vi "Main.vi"() -> ()   [LabVIEW 2024]
uses:
  <vilib>/userDefined/High Color/IMAQdx.ctl
  <vilib>/vision/Image Controls.llb/IMAQ Image.ctl
  <vilib>/vision/driver/NI_Vision_Acquisition_Software.lvlib
panel:
  in  "Exit Application":bool caption="Click to terminate the application"
  in  "Tab Control":enum32{"Page 1", "Page 2", "Page 3", "Page 4"}(tab)
  in  "OK Button":bool
  out "Image Display":T1(plugin-control)
  in  "Settings Button":bool
  in  "Add user":bool
  out "Current VI":path
  in  "Back to userpage":bool
  out "Image Display 2":T1(plugin-control)
  in  "OK Button 2":bool
  in  "String":string
  in  "String 2":string
  # "Processing..."
  # "Welcome to control panel"
  # "Now you can chose what you want to do"
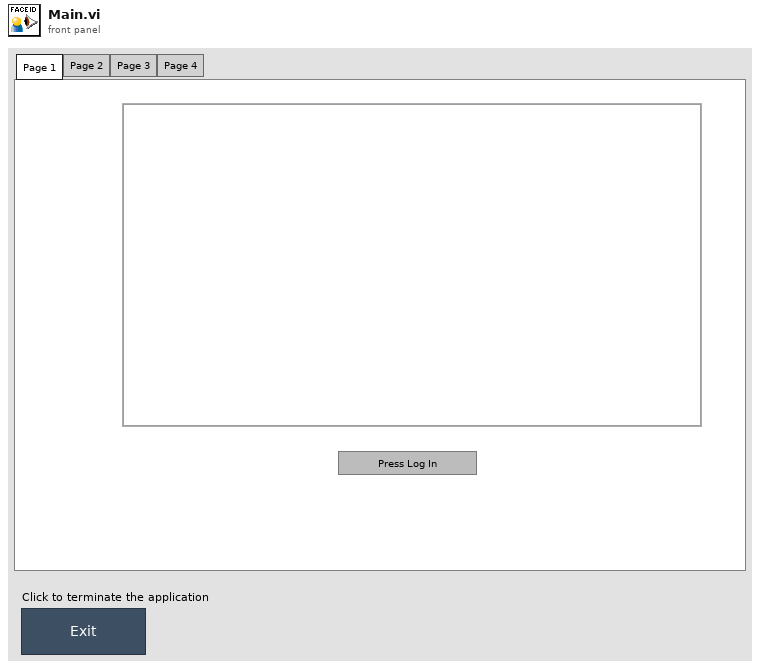
[diagram p1: front panel]
types:
  T1 = typedef "IMAQ Image.ctl" = refnum<image>
  T2 = enum32{"Invalid", "Standard", "Closed", "Hidden", "Minimized", "Maximized"}
  T3 = enum32{"invalid app kind", "Development System", "Run Time System", "Student Edition", "Embedded LabVIEW", "Evaluation", "Custom"}
  T4 = typedef "IMAQdx.ctl" = refnum<k21>
  T5 = cluster{"Core":cluster{"Current VI Reference":refnum<vi>, "Close Panel on Exit?":bool}, "New Image":T1, "IMAQdx Session":T4, "Img Path":string}
  T6 = cluster{"Current VI Reference":refnum<vi>, "Close Panel on Exit?":bool}
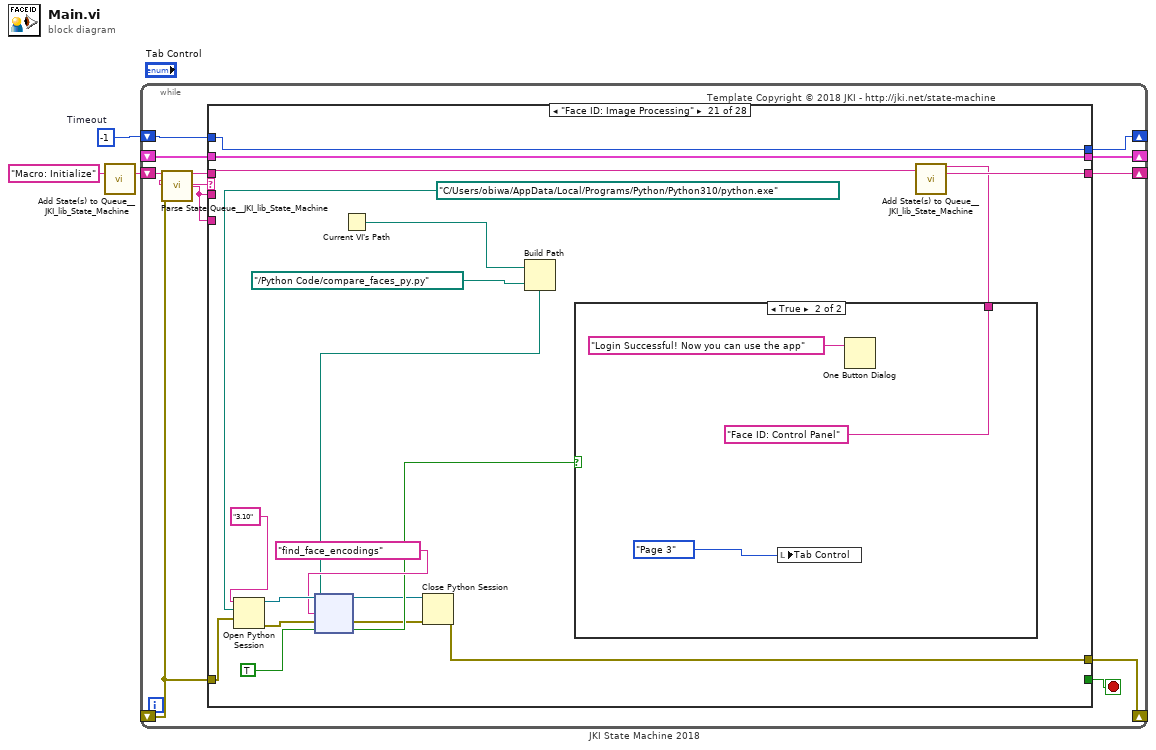
[diagram p0: block diagram]
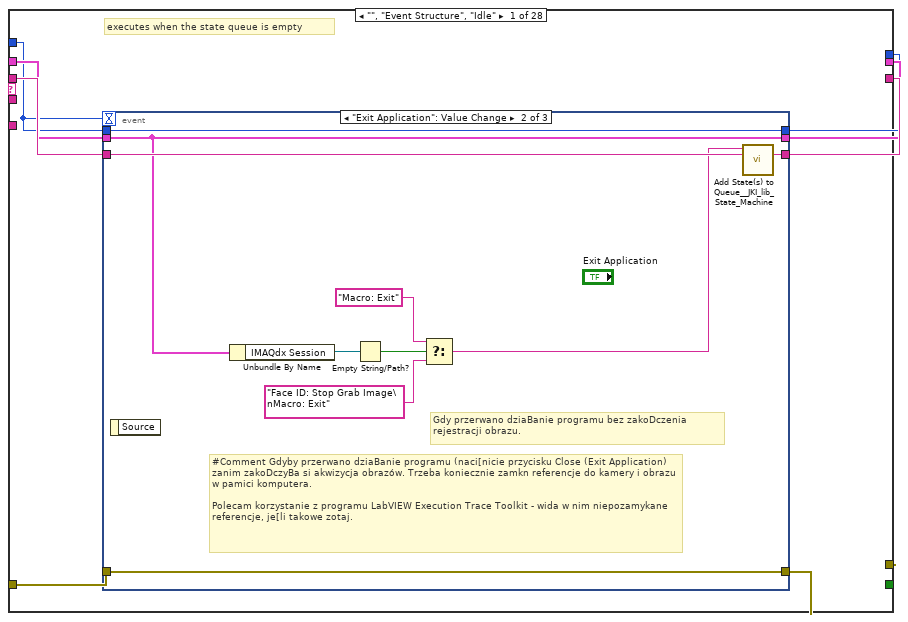
[diagram p2: hidden frame]
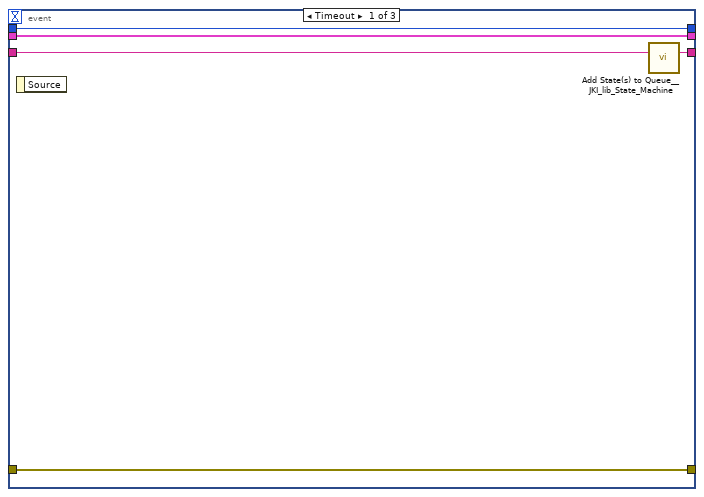
[diagram p3: hidden frame]
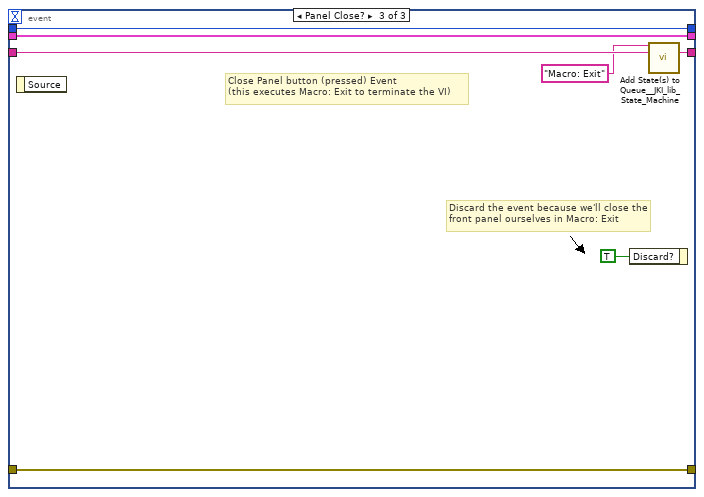
[diagram p4: hidden frame]
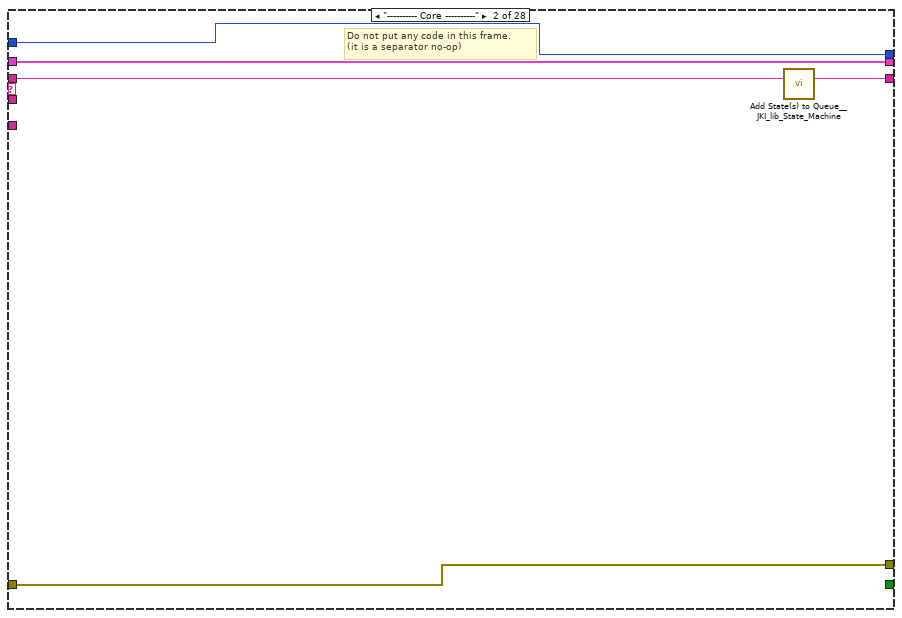
[diagram p5: hidden frame]
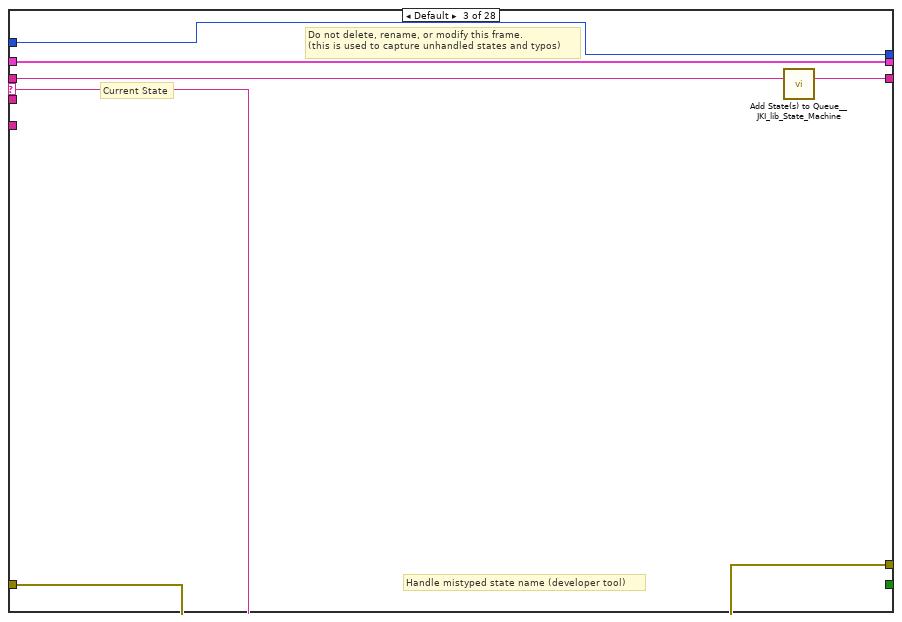
[diagram p6: hidden frame]
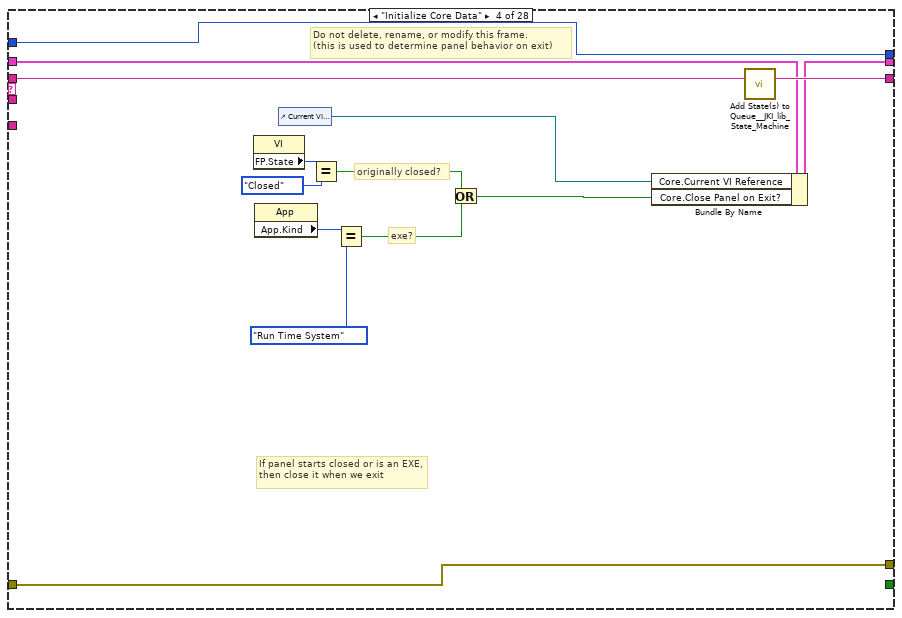
[diagram p7: hidden frame]
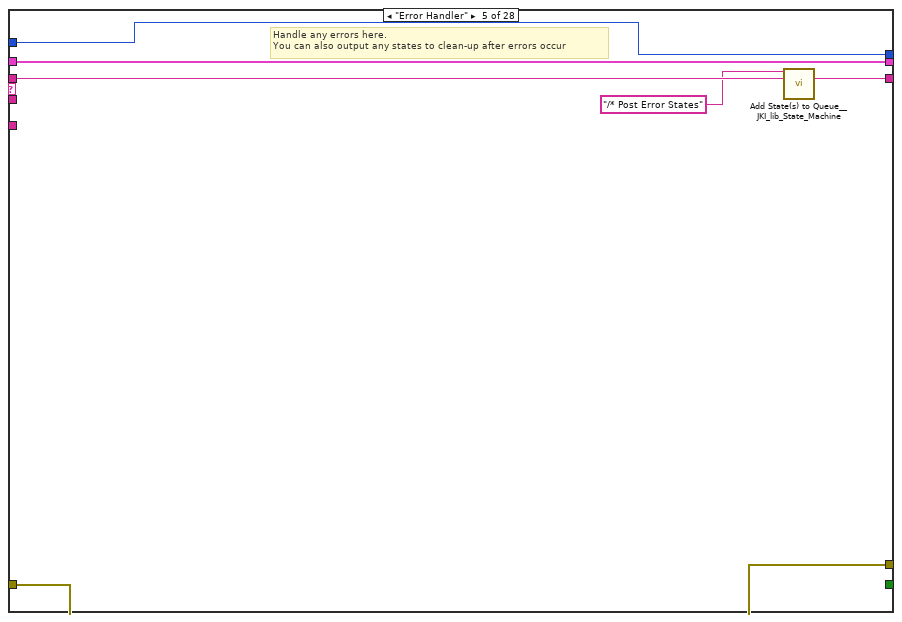
[diagram p8: hidden frame]
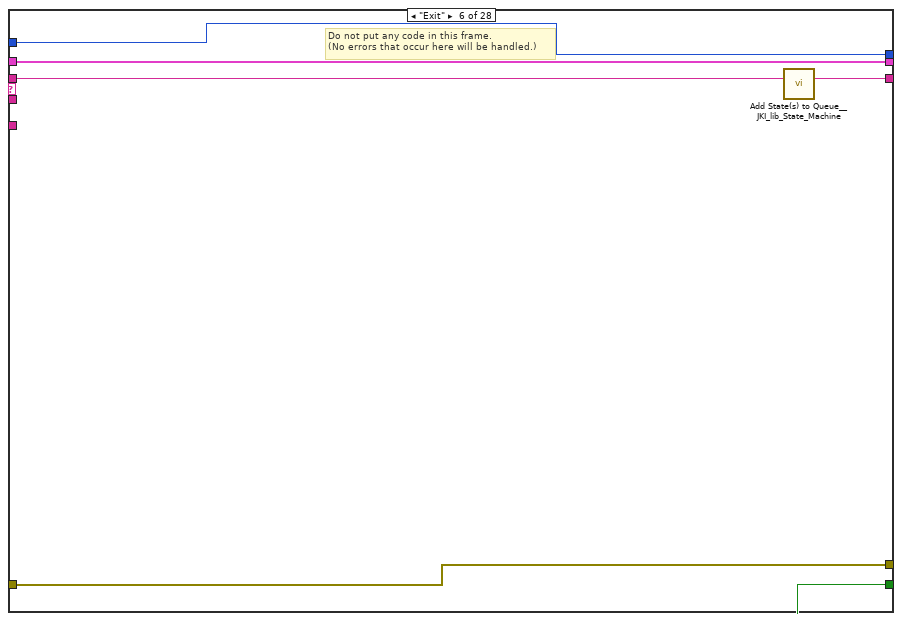
[diagram p9: hidden frame]
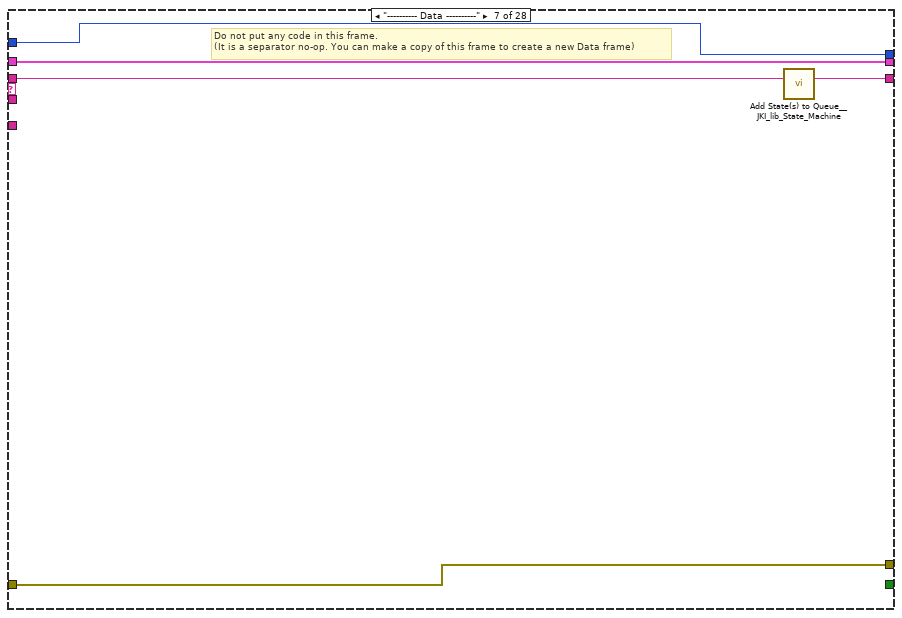
[diagram p10: hidden frame]
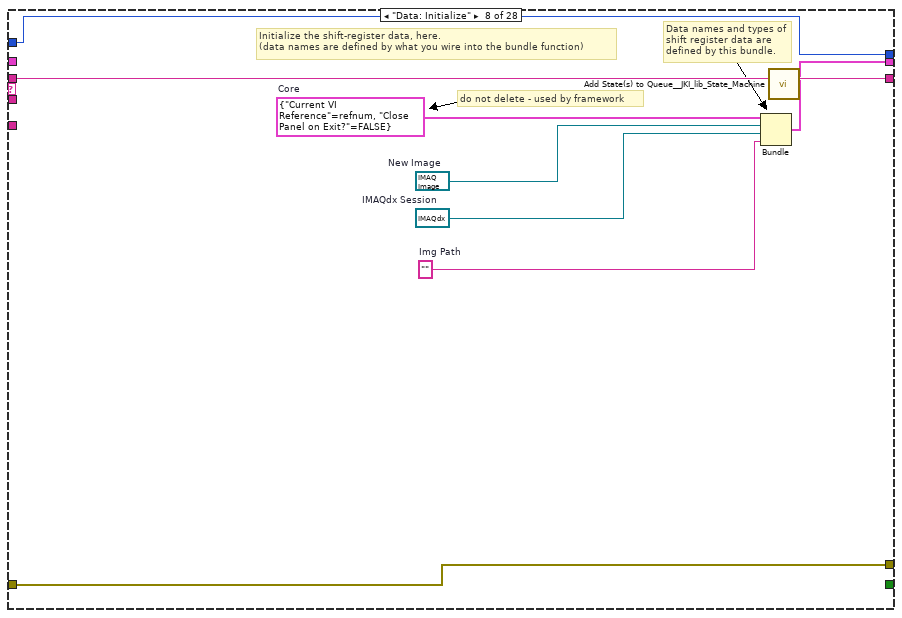
[diagram p11: hidden frame]
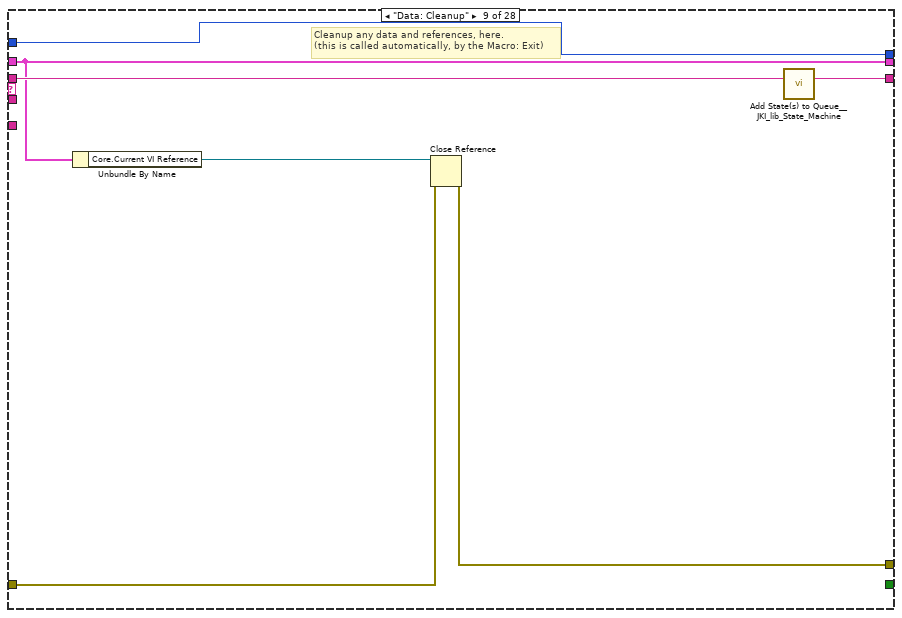
[diagram p12: hidden frame]
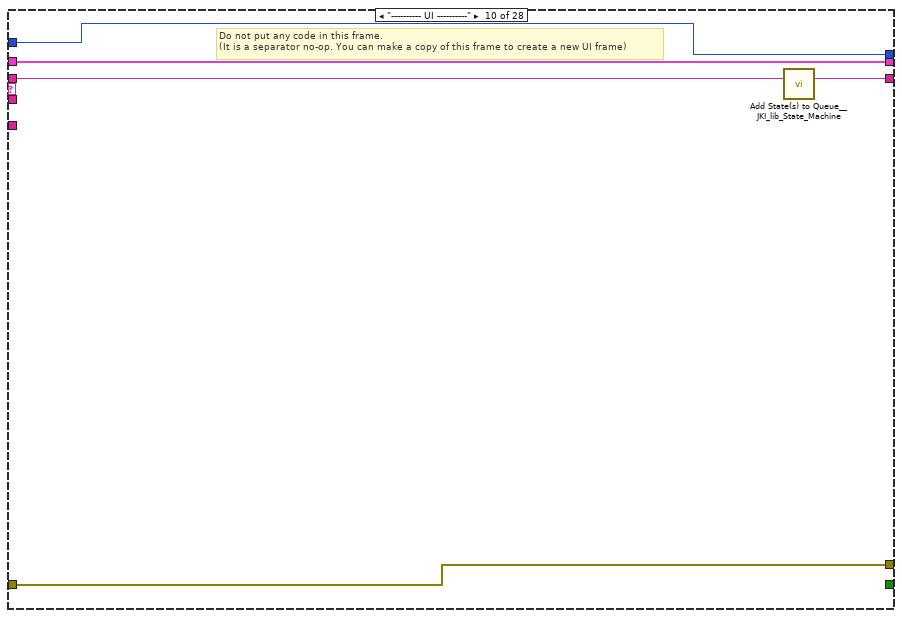
[diagram p13: hidden frame]
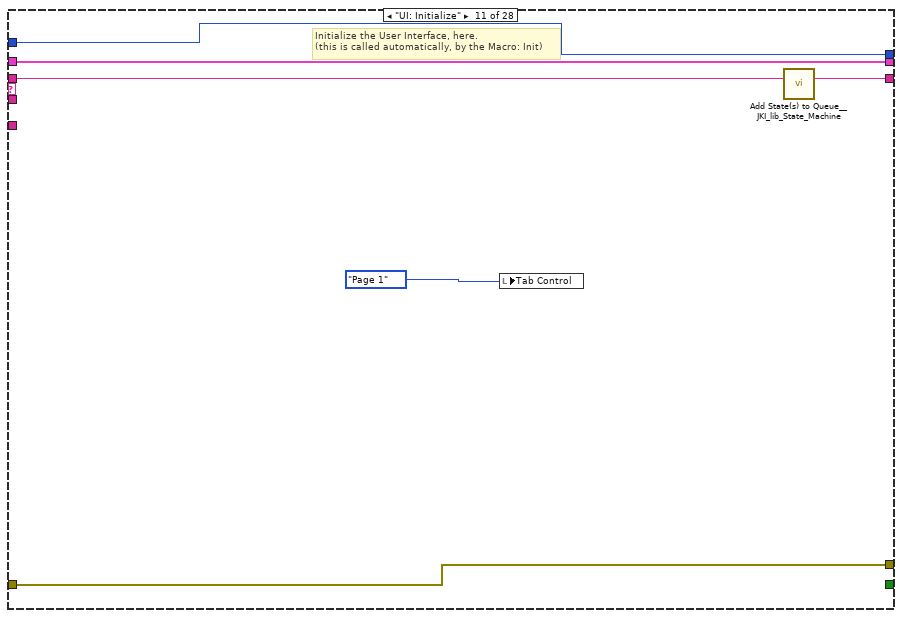
[diagram p14: hidden frame]
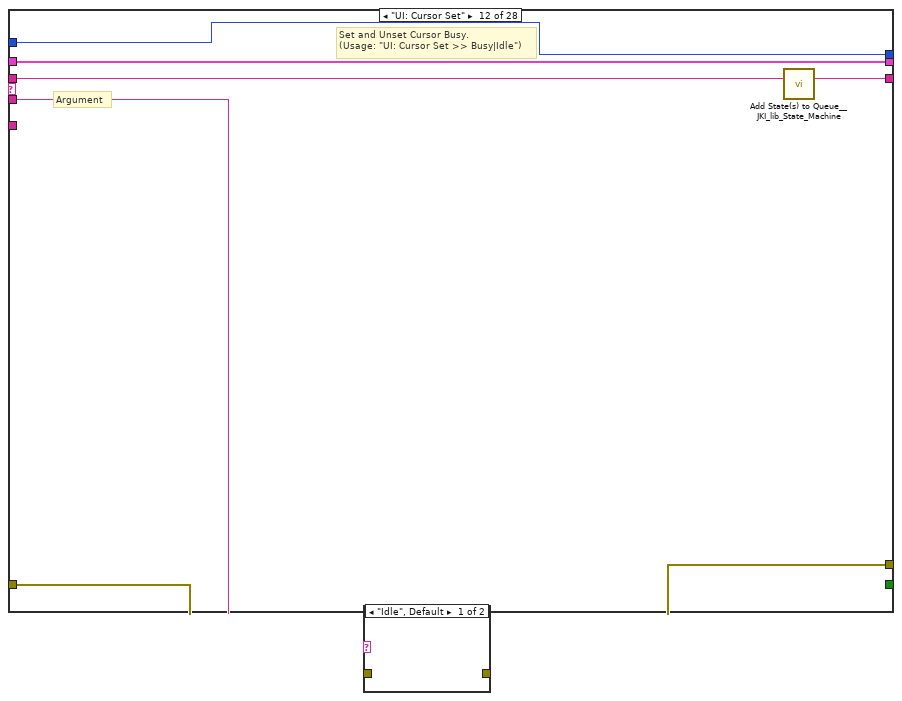
[diagram p15: hidden frame]
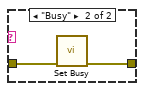
[diagram p16: hidden frame]
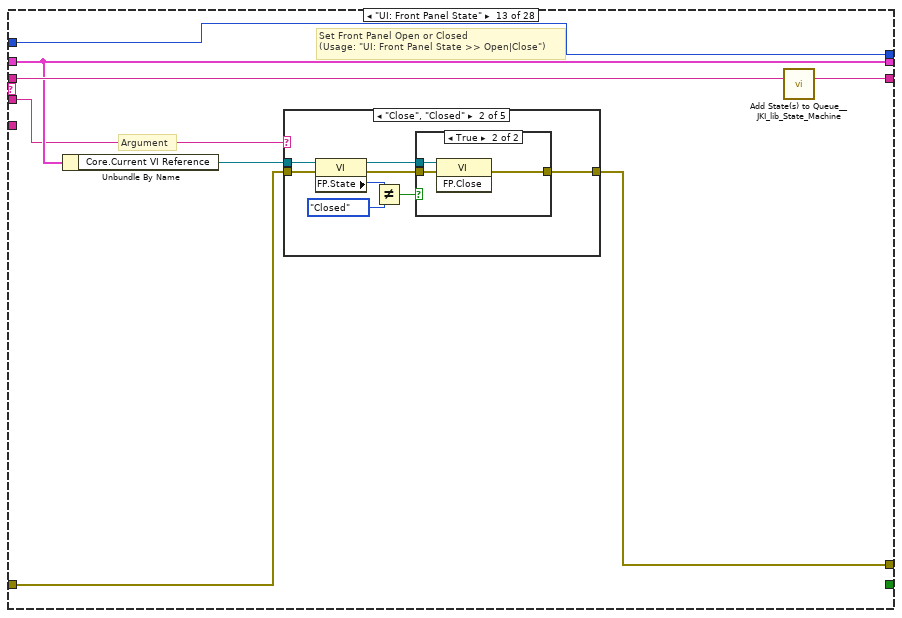
[diagram p17: hidden frame]
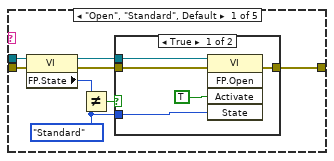
[diagram p18: hidden frame]
diagram:
  w1 = -1  # Timeout
  n1 = call <vilib>:"Add State(s) to Queue__JKI_lib_State_Machine.vi"("State(s) in (\"\")"="Macro: Initialize") -> ("States Out"=w3:string)  [unwired: 14 in]
  n2 = while "JKI State Machine 2018" {
    shift-right: [w9] -> _
    shift-left: _ -> [w8]
    shift-right: [w12] -> _
    shift-left: _ -> [w7]
    shift-right: [w11] -> _
    shift-left: w3 -> [w13]
    shift-right: [w5] -> _
    shift-left: w1 -> [w6]
    stop <- w10 stop-if-true
    # "Template Copyright © 2018 JKI - http://jki.net/state-machine"
    n3 = call <vilib>:"Parse State Queue__JKI_lib_State_Machine.vi"("State Queue"=w13, "Error In (no error)"=w7) -> ("Remaining States"=w14:string, "Current State"=w15:string, "Arguments"=w4:string)  [unwired: 11 in]
    n4 = case shown="\"Face ID: Image Processing\"" w15 {
      selector: w15 -> [_ _ w52 _ _ _ _ _ _ _ _ _ _ _ _ _ _ _ _ _ _ _ _ _ _ _ _ _]
      tunnel: w14 -> [w23 w50 w56 w76 w83 w89 w94 w103 w110 w115 w121 w128 w140 w210 w216 w227 w232 w240 w280 w301 w319 w332 w343 w348 w351 w360 w401 w419]
      tunnel: w4 -> [_ _ _ _ _ _ _ _ _ _ _ w123 w134 _ _ _ _ _ _ _ _ _ _ _ _ _ _ _]
      tunnel: w8 -> [w21 w47 w54 w69 w80 w84 w91 _ w105 w112 w119 w126 w136 w207 w213 w224 w229 w233 w277 w290 w317 w328 w344 w347 w352 w355 w402 w420]
      tunnel: [w20 w48 w58 w73 errorcluster {"status"=FALSE, "code"=0, "source"=""} ("error out") w87 w92 w100 w106 w113 w118 w124 w137 w208 w214 w225 w230 w242 w272 w287 w307 w337 w342 w346 w350 w358 w399 w418] -> w12
      tunnel: w7 -> [w19 w48 w57 w73 w79 w87 w92 w100 w107 w113 w118 w125 w138 w208 w214 w225 w230 w241 w273 w294 w315 w337 w342 w346 w350 w359 w400 _]
      tunnel: [w22 w49 w55 w75 w82 w88 w93 w102 w109 w114 w120 w127 w139 w209 w215 w226 w231 w250 w279 w300 w318 w333 w343 w348 w351 w357 w404 w415] -> w11
      tunnel: [_ _ _ _ _ TRUE _ _ _ _ _ _ _ _ _ _ _ _ _ _ _ _ _ _ _ _ _ _] -> w10
      tunnel: [w18 w47 w54 w74 w80 w84 w91 w101 w105 w112 w119 w126 w136 w207 w213 w224 w229 w234 w278 w291 w317 w328 w344 w347 w352 w354 w403 w416] -> w9
      tunnel: w6 -> [w17 w46 w51 w63 w77 w85 w90 w96 w104 w111 w117 w122 w133 w206 w211 w218 w228 w235 w276 _ w320 w338 w345 w349 w353 w361 w410 _]
      tunnel: [w16 w46 w51 w63 w77 w85 w90 w96 w104 w111 w117 w122 w133 w206 w211 w218 w228 w236 w276 -1 ("Timeout") w320 w338 w345 w349 w353 w356 w410 -1 ("Timeout")] -> w5
      tunnel: w4 -> [_ _ _ _ _ _ _ _ _ _ _ _ _ _ _ _ _ _ _ _ _ _ _ _ _ _ _ _]
      frame "", "Event Structure", "Idle" {
        # "executes when the state queue is empty"
        n5 = event shown="[1] \"Exit Application\": Value Change" {
          selector: _ -> [_ _ _]
          dyn-events: _ -> [_ _ _]
          timeout: w17 -> [_ _ _]
          tunnel: w23 -> [w28 w38 w45]
          tunnel: [w27 w37 w44] -> w22
          tunnel: w21 -> [w25 w33 w42]
          tunnel: [w26 w36 w43] -> w20
          tunnel: w19 -> [w26 w36 w43]
          tunnel: [w25 w33 w42] -> w18
          tunnel: w17 -> [w24 w35 w39]
          tunnel: [w24 w35 w39] -> w16
          event Timeout {
            n6 = event-data() -> ()  [unwired: 1 in, 1 out]
            n7 = call <vilib>:"Add State(s) to Queue__JKI_lib_State_Machine.vi"("State(s) in (\"\")"=w28) -> ("States Out"=w27:string)  [unwired: 14 in]
          }
          event "Exit Application": Value Change {
            # "Gdy przerwano dziaBanie programu bez zakoDczenia rejestracji obrazu."
            # "#Comment Gdyby przerwano dziaBanie programu (naci[nicie przycisku Close (Exit Application) zanim zakoDczyBa si akwizycja obrazów. Trzeba koniecznie zamkn referencje do kamery i obrazu w pamici komputera.\n\nPolecam korzystanie z programu LabVIEW Execution Trace Toolkit - wida w nim niepozamykane referencje, je[li takowe zotaj."
            n8 = event-data() -> ()  [unwired: 1 in, 1 out]
            n9 = Unbundle By Name(w33) -> ("IMAQdx Session"=w34:T4)
            n10 = Empty String/Path?(string/path=w34) -> (empty?=w32:bool)
            n11 = Select(t="Macro: Exit", s=w32, f="Face ID: Stop Grab Image\nMacro: Exit") -> (s? t:f=w31:string)
            n12 = call <vilib>:"Add State(s) to Queue__JKI_lib_State_Machine.vi"("State(s) in Front (\"\")"=w31, "State(s) in (\"\")"=w38) -> ("States Out"=w37:string)  [unwired: 13 in]
          }
          event Panel Close? {
            # "Discard the event because we'll close the front panel ourselves in Macro: Exit"
            # "Close Panel button (pressed) Event\n(this executes Macro: Exit to terminate the VI)"
            n13 = event-data() -> ()  [unwired: 1 in, 1 out]
            n14 = event-data("Discard?"=TRUE) -> ()  [unwired: 1 in, 1 out]
            n15 = call <vilib>:"Add State(s) to Queue__JKI_lib_State_Machine.vi"("State(s) in Front (\"\")"="Macro: Exit", "State(s) in (\"\")"=w45) -> ("States Out"=w44:string)  [unwired: 13 in]
          }
        }
      }
      frame "---------- Core ----------" {
        # "Do not put any code in this frame.\n(it is a separator no-op)"
        n16 = call <vilib>:"Add State(s) to Queue__JKI_lib_State_Machine.vi"("State(s) in (\"\")"=w50) -> ("States Out"=w49:string)  [unwired: 14 in]
      }
      frame Default {
        w61 = 42 items=["No error", "Argument error", "Memory is full", "Out of zone", "End of file", "File already open", "Generic file I/O error", "File not found", "File permission error", "Disk is full", "Duplicate path", "Too many files open", "System feature not enabled", "Resource file not found", "Cannot add resource", "Resource not found", "Image not found", "Image memory error", "Pen does not exist", "Config type invalid", "Config token not found", "Config parse error", "Config memory error", "Bad external code format", "Bad external code offset", "External code not present", "Null window", "Destroy window error", "Null menu", "Print aborted", "Bad print record", "Print driver error", "Windows error during printing", "Memory error during printing", "Print dialog error", "Generic print error", "Invalid device refnum", "Device not found", "Device parameter error", "Device unit error", "Cannot open device", "Device call aborted", "Generic error", "Cancelled by user", "Object ID too low", "Object ID too high", "Object not in heap", "Unknown heap", "Unknown object (invalid DefProc)", "Unknown object (DefProc not in table)", "Message out of range", "Invalid (null) method", "Unknown message", "Manager call not supported", "Bad address", "Network operation in progress", "Network operation timed out", "Connection is busy", "Network attribute not supported", "Network error", "Address in use", "System out of memory", "Connection aborted", "Connection refused", "Not connected", "Already connected", "Connection closed", "Initialization error (interapplication manager)", "Bad occurrence", "Wait on unbound occurrence handler", "Occurrence queue overflow", "Datalog type conflict", "Unused", "Unrecognized type (interapplication manager)", "Memory corrupt", "Failed to make temporary DLL", "Old CIN version", "Drag socket not found", "Failed to load drop-object", "Failed to register OLE object", "Failed to release OLE object", "Format specifier type mismatch", "Unknown format specifier", "Too few format specifiers", "Too many format specifiers", "Scan failed", "Newer CIN version", "Error converting to variant", "Runtime menu error", "Password tampered", "Variant attribute not found", "Incompatible variant data type", "Event data is not available", "Event Store is not present", "Occurrence is not found", "Event Queue is not created", "Event info is not available", "Refnum passed is NULL", "Error retrieving Class GUID", "Error retrieving CoClass GUID", "Error retrieving TypeLib GUID.", "Bad built application magic bytes.", "Specific driver is different from the specific driver associated with the Logical Name.", "There is no session opened to the class driver.", "Max Error", "MAX - Error with config objects", "MAX - Error loading configuration", "MAX - Group not supported"]
        # "Current State"
        # "Do not delete, rename, or modify this frame.\n(this is used to capture unhandled states and typos)"
        # "Handle mistyped state name (developer tool)"
        n17 = Format Into String(format string="Software Exception: Unhandled State \"%s\"." ("message"), error in=w57, w52) -> (resulting string=w60:string, error out=w59:errorcluster)  [unwired: 1 in]
        n18 = call <vilib>:"Error Cluster From Error Code.vi"("show call chain? (False)"=TRUE, "error in (no error)"=w59, "error message (\"\")"=w60, "error code (0)"=w61) -> ("error out"=w58:errorcluster)  [unwired: 5 in]
        n19 = call <vilib>:"Add State(s) to Queue__JKI_lib_State_Machine.vi"("State(s) in (\"\")"=w56) -> ("States Out"=w55:string)  [unwired: 14 in]
      }
      frame "Initialize Core Data" {
        # "Do not delete, rename, or modify this frame.\n(this is used to determine panel behavior on exit)"
        # "originally closed?"
        # "exe?"
        # "If panel starts closed or is an EXE, then close it when we exit"
        n20 = property class="VI"() -> ("FP.State"=w66:T2)  [unwired: 2 in, 2 out]
        n21 = property class="App"() -> ("App.Kind"=w72:T3)  [unwired: 2 in, 2 out]
        n22 = control-ref of="Current VI Reference"() -> (w67:refnum<vi>)
        n23 = Equal?(x=w66, y=T2."Closed" ("Front Panel Window:State")) -> (x = y?=w64:bool)
        n24 = Equal?(x=w72, y=T3."Run Time System" ("Application:Kind")) -> (x = y?=w70:bool)
        n25 = Or(x=w64, y=w70) -> (x .or. y?=w68:bool)
        n26 = Bundle By Name(cluster=w69, "Core.Current VI Reference"=w67, "Core.Close Panel on Exit?"=w68) -> (w74:T5)
        n27 = call <vilib>:"Add State(s) to Queue__JKI_lib_State_Machine.vi"("State(s) in (\"\")"=w76) -> ("States Out"=w75:string)  [unwired: 14 in]
      }
      frame "Error Handler" {
        # "Unhandled Error -- Display it"
        # "Handle any errors here.\nYou can also output any states to clean-up after errors occur"
        # "Clear error"
        n28 = call <vilib>:"General Error Handler.vi"("error in (no error)"=w79) -> ()  [unwired: 10 in, 5 out]
        n29 = call <vilib>:"Add State(s) to Queue__JKI_lib_State_Machine.vi"("State(s) in Front (\"\")"="/* Post Error States", "State(s) in (\"\")"=w83) -> ("States Out"=w82:string)  [unwired: 13 in]
      }
      frame "Exit" {
        # "Do not put any code in this frame.\n(No errors that occur here will be handled.)"
        n30 = call <vilib>:"Add State(s) to Queue__JKI_lib_State_Machine.vi"("State(s) in (\"\")"=w89) -> ("States Out"=w88:string)  [unwired: 14 in]
      }
      frame "---------- Data ----------" {
        # "Do not put any code in this frame.\n(It is a separator no-op. You can make a copy of this frame to create a new Data frame)"
        n31 = call <vilib>:"Add State(s) to Queue__JKI_lib_State_Machine.vi"("State(s) in (\"\")"=w94) -> ("States Out"=w93:string)  [unwired: 14 in]
      }
      frame "Data: Initialize" {
        w95 = ""  # Img Path
        w97 = T1 refnum  # New Image
        w98 = T4 refnum  # IMAQdx Session
        w99 = T6 {"Current VI Reference"=refnum, "Close Panel on Exit?"=FALSE}  # Core
        # "do not delete - used by framework"
        # "Data names and types of shift register data are defined by this bundle."
        # "Initialize the shift-register data, here.\n(data names are defined by what you wire into the bundle function)"
        n32 = Bundle("Core"=w99, "New Image"=w97, "IMAQdx Session"=w98, "Img Path"=w95) -> (w101:T5)  [unwired: 1 in]
        n33 = call <vilib>:"Add State(s) to Queue__JKI_lib_State_Machine.vi"("State(s) in (\"\")"=w103) -> ("States Out"=w102:string)  [unwired: 14 in]
      }
      frame "Data: Cleanup" {
        # "Cleanup any data and references, here.\n(this is called automatically, by the Macro: Exit)"
        n34 = Unbundle By Name(w105) -> ("Core.Current VI Reference"=w108:refnum<vi>)
        n35 = Close Reference(reference=w108, error in (no error)=w107) -> (error out=w106:errorcluster)
        n36 = call <vilib>:"Add State(s) to Queue__JKI_lib_State_Machine.vi"("State(s) in (\"\")"=w110) -> ("States Out"=w109:string)  [unwired: 14 in]
      }
      frame "---------- UI ----------" {
        # "Do not put any code in this frame.\n(It is a separator no-op. You can make a copy of this frame to create a new UI frame)"
        n37 = call <vilib>:"Add State(s) to Queue__JKI_lib_State_Machine.vi"("State(s) in (\"\")"=w115) -> ("States Out"=w114:string)  [unwired: 14 in]
      }
      frame "UI: Initialize" {
        # "Initialize the User Interface, here.\n(this is called automatically, by the Macro: Init)"
        n38 = local write "Tab Control"(enum32{"Page 1", "Page 2", "Page 3", "Page 4"}."Page 1" ("Tab Control")) -> ()
        n39 = call <vilib>:"Add State(s) to Queue__JKI_lib_State_Machine.vi"("State(s) in (\"\")"=w121) -> ("States Out"=w120:string)  [unwired: 14 in]
      }
      frame "UI: Cursor Set" {
        # "Argument"
        # "Set and Unset Cursor Busy.\n(Usage: \"UI: Cursor Set >> Busy|Idle\")"
        n40 = case shown="\"Idle\", Default" w123 {
          tunnel: w125 -> [w130 w132]
          tunnel: [w129 w131] -> w124
          frame "Idle", Default {
            n41 = call <vilib>:"Unset Busy.vi"("error in (no error)"=w130) -> ("error out"=w129:errorcluster)  [unwired: 10 in]
          }
          frame "Busy" {
            n42 = call <vilib>:"Set Busy.vi"("error in (no error)"=w132) -> ("error out"=w131:errorcluster)  [unwired: 9 in, 1 out]
          }
        }
        n43 = call <vilib>:"Add State(s) to Queue__JKI_lib_State_Machine.vi"("State(s) in (\"\")"=w128) -> ("States Out"=w127:string)  [unwired: 14 in]
      }
      frame "UI: Front Panel State" {
        # "Argument"
        # "Set Front Panel Open or Closed\n(Usage: \"UI: Front Panel State >> Open|Close\")"
        n44 = Unbundle By Name(w136) -> ("Core.Current VI Reference"=w135:refnum<vi>)
        n45 = case shown="\"Close\", \"Closed\"" w134 {
          tunnel: w138 -> [w146 w161 w172 w185 w198]
          tunnel: [w148 w162 w174 w187 w200] -> w137
          tunnel: w135 -> [w147 w159 w173 w186 w199]
          frame "Open", "Standard", Default {
            w141 = T2."Standard" ("State")
            n46 = property class="VI"(reference=w147, error in=w146) -> (reference out=w144:refnum<vi>, error out=w145:errorcluster, "FP.State"=w143:T2)
            n47 = Not Equal?(x=w143, y=w141) -> (x != y?=w142:bool)
            n48 = case shown="True" w142 {
              tunnel: [w152 w154] -> w148
              tunnel: w145 -> [w151 w154]
              tunnel: w144 -> [w150 _]
              tunnel: w141 -> [w149 _]
              frame True {
                n49 = invoke class="VI" method="FP.Open"(reference=w150, error in=w151, "Activate"=TRUE, "State"=w149) -> (error out=w152:errorcluster)  [unwired: 1 in, 4 out]
              }
              frame False {
              }
            }
          }
          frame "Close", "Closed" {
            n50 = property class="VI"(reference=w159, error in=w161) -> (reference out=w158:refnum<vi>, error out=w160:errorcluster, "FP.State"=w156:T2)
            n51 = Not Equal?(x=w156, y=T2."Closed" ("Front Panel Window:State")) -> (x != y?=w155:bool)
            n52 = case shown="True" w155 {
              tunnel: [w163 w166] -> w162
              tunnel: w160 -> [w163 w165]
              tunnel: w158 -> [_ w164]
              frame False {
              }
              frame True {
                n53 = invoke class="VI" method="FP.Close"(reference=w164, error in=w165) -> (error out=w166:errorcluster)  [unwired: 1 in, 2 out]
              }
            }
          }
          frame "Hidden", "Hide" {
            w167 = T2."Hidden" ("State")
            n54 = property class="VI"(reference=w173, error in=w172) -> (reference out=w170:refnum<vi>, error out=w171:errorcluster, "FP.State"=w169:T2)
            n55 = Not Equal?(x=w169, y=w167) -> (x != y?=w168:bool)
            n56 = case shown="True" w168 {
              tunnel: [w178 w179] -> w174
              tunnel: w171 -> [w177 w179]
              tunnel: w170 -> [w176 _]
              tunnel: w167 -> [w175 _]
              frame True {
                n57 = invoke class="VI" method="FP.Open"(reference=w176, error in=w177, "State"=w175) -> (error out=w178:errorcluster)  [unwired: 2 in, 4 out]
              }
              frame False {
              }
            }
          }
          frame "Minimize", "Minimized" {
            w180 = T2."Minimized" ("State")
            n58 = property class="VI"(reference=w186, error in=w185) -> (reference out=w183:refnum<vi>, error out=w184:errorcluster, "FP.State"=w182:T2)
            n59 = Not Equal?(x=w182, y=w180) -> (x != y?=w181:bool)
            n60 = case shown="True" w181 {
              tunnel: [w191 w192] -> w187
              tunnel: w184 -> [w190 w192]
              tunnel: w183 -> [w189 _]
              tunnel: w180 -> [w188 _]
              frame True {
                n61 = invoke class="VI" method="FP.Open"(reference=w189, error in=w190, "State"=w188) -> (error out=w191:errorcluster)  [unwired: 2 in, 4 out]
              }
              frame False {
              }
            }
          }
          frame "Maximize", "Maximized" {
            w193 = T2."Maximized" ("State")
            n62 = property class="VI"(reference=w199, error in=w198) -> (reference out=w196:refnum<vi>, error out=w197:errorcluster, "FP.State"=w195:T2)
            n63 = Not Equal?(x=w195, y=w193) -> (x != y?=w194:bool)
            n64 = case shown="True" w194 {
              tunnel: [w204 w205] -> w200
              tunnel: w197 -> [w203 w205]
              tunnel: w196 -> [w202 _]
              tunnel: w193 -> [w201 _]
              frame True {
                n65 = invoke class="VI" method="FP.Open"(reference=w202, error in=w203, "State"=w201) -> (error out=w204:errorcluster)  [unwired: 2 in, 4 out]
              }
              frame False {
              }
            }
          }
        }
        n66 = call <vilib>:"Add State(s) to Queue__JKI_lib_State_Machine.vi"("State(s) in (\"\")"=w140) -> ("States Out"=w139:string)  [unwired: 14 in]
      }
      frame "---------- Macro ----------" {
        # "Do not put any code in this frame.\n(It is a separator no-op. You can make a copy of this frame to create a new Macro frame)"
        n67 = call <vilib>:"Add State(s) to Queue__JKI_lib_State_Machine.vi"("State(s) in (\"\")"=w210) -> ("States Out"=w209:string)  [unwired: 14 in]
      }
      frame "Macro: Initialize" {
        w212 = "Data: Initialize\nInitialize Core Data\nUI: Initialize\nUI: Front Panel State >> Open\nFace ID: Initialize Grab Image"  # Data: Initialize Initialize Core Data UI: Initialize UI: Front Panel State >> Open Face ID: Initialize Grab Image
        # "Initialization Macro\n(This is called once, when the VI starts)"
        n68 = call <vilib>:"Add State(s) to Queue__JKI_lib_State_Machine.vi"("State(s) in Front (\"\")"=w212, "State(s) in (\"\")"=w216) -> ("States Out"=w215:string)  [unwired: 13 in]
      }
      frame "Macro: Exit" {
        # "Exit Macro\n(This is called once, when the VI exits)"
        n69 = Unbundle By Name(w224) -> ("Core.Close Panel on Exit?"=w223:bool)
        n70 = Select(t="UI: Front Panel State >> Close", s=w223, f="") -> (s? t:f=w220:string)
        n71 = call <vilib>:"Add State(s) to Queue__JKI_lib_State_Machine.vi"("State(s) in (\"\")"=w220, "State(s) at Back (\"\")"="Data: Cleanup\nExit") -> ("States Out"=w219:string)  [unwired: 13 in]
        n72 = call <vilib>:"Add State(s) to Queue__JKI_lib_State_Machine.vi"("State(s) in Front (\"\")"=w219, "State(s) in (\"\")"=w227) -> ("States Out"=w226:string)  [unwired: 13 in]
      }
      frame "---------- Face ID ----------" {
        # "Template Separator\n(You can make a copy of, or modify, this frame)"
        n73 = call <vilib>:"Add State(s) to Queue__JKI_lib_State_Machine.vi"("State(s) in (\"\")"=w232) -> ("States Out"=w231:string)  [unwired: 14 in]
      }
      frame "Face ID: Initialize Grab Image" {
        # "#Comment BazowaBem na przykBadzie Acquire Most Recent Image.vi z Find Examples"
        # "1 Wyszukuje dostpne kamery\n2 Okno dialogowe wyboru kamery (przez u|ytkownika). Mo|na usun lub obj Diagram Disable Structure, je[i niepotrzebne.\n3 Konfiguracja kamery\n4 Konfiguracja akwizycji obrazów"
        # "2"
        # "1"
        n74 = call "List Available Cameras.vi"("error in"=w241) -> ("error out"=w247:errorcluster, "VendorName"=w248:string[], "Available Cameras"=w249:string[])  [unwired: 8 in]
        n75 = call "Select Camera Dialog.vi"("error in (no error)"=w247, "Vendor Name"=w248, "Camera Name"=w249) -> ("error out"=w243:errorcluster, "No camera?"=w246:bool, "Interface Name"=w245:string)  [unwired: 6 in]
        n76 = case shown="False" w246 {
          tunnel: w245 -> [w261 _]
          tunnel: [w259 T4 refnum ("Session Out")] -> w244
          tunnel: w243 -> [w257 w266]
          tunnel: [w256 w266] -> w242
          tunnel: w240 -> [w255 _]
          tunnel: [w255 w264] -> w239
          tunnel: [w253 T1 refnum ("New Image")] -> w238
          tunnel: ["Face ID: Grab Image" ("Remaining States") w264] -> w237
          tunnel: [10 w263] -> w236
          tunnel: w235 -> [_ w263]
          frame False {
            w262 = u32 5  # Number of Buffers
            # "{eby nam nie zatrzymaB si w \", \"Event Structure\", \"Idle\" generujemy Timeout"
            # "Musimy stworzy referencj dla przechowywania obrazu w pamici komputera."
            # "4"
            # "3"
            n77 = call <vilib>:"IMAQdx Open Camera.vi"("error in"=w257, "Session In"=w261) -> ("error out"=w258:errorcluster, "Session Out"=w260:T4)  [unwired: 1 in, 7 out]
            n78 = call <vilib>:"IMAQdx Configure Grab.vi"("error in"=w258, "Number of Buffers"=w262, "Session In"=w260) -> ("error out"=w256:errorcluster, "Session Out"=w259:T4)  [unwired: 7 in]
            n79 = call "IMAQ Create"("Image Name"="Acquire Most Recent Image") -> ("New Image"=w253:T1)  [unwired: 3 in, 2 out]
          }
          frame True {
            w264 = ""
            # "Kasujemy kolejne stany.\n! I tak \"idzie\" do \"Error Handler\"."
            # "Generuje bBd: -1074360311"
            # "Camera not found"
          }
        }
        n80 = Bundle By Name(cluster=w233, "New Image"=w238, "IMAQdx Session"=w244) -> (w234:T5)
        n81 = call <vilib>:"Add State(s) to Queue__JKI_lib_State_Machine.vi"("State(s) in Front (\"\")"=w237, "State(s) in (\"\")"=w239) -> ("States Out"=w250:string)  [unwired: 13 in]
      }
      frame "Face ID: Grab Image" {
        # "Rejestrujemy obrazy...\nPrzetwarzanie obrazów mo|na doda tutaj albo stworzy osobny stan."
        n82 = Unbundle By Name(w277) -> ("IMAQdx Session"=w275:T4, "New Image"=w274:T1)
        n83 = call "Take Image Case Struct.vi"("error in (no error)"=w273, "OK Button"="OK Button", "Image In"=w274, "Session In"=w275) -> ("error out"=w272:errorcluster, "f"=w270:string, "Image Out"=w269:T1, "Session Out"=w271:T4)  [unwired: 4 in]
        "Image Display" <- w269
        n84 = Bundle By Name(cluster=w277, "IMAQdx Session"=w271, "New Image"=w269) -> (w278:T5)
        n85 = call <vilib>:"Add State(s) to Queue__JKI_lib_State_Machine.vi"("State(s) in Front (\"\")"=w270, "State(s) in (\"\")"=w280) -> ("States Out"=w279:string)  [unwired: 13 in]
      }
      frame "Face ID: Stop Grab Image" {
        # "WyBczamy Timeout"
        # "Sukces! Wykryli[my twarz, lecimy dalej!"
        n86 = Current VI's Path() -> (path=w285:path)
        n87 = Unbundle By Name(w290) -> ("New Image"=w286:T1, "IMAQdx Session"=w295:T4)
        n88 = call <vilib>:"IMAQdx Stop Acquisition.vi"("error in"=w294, "Session In"=w295) -> ("error out"=w299:errorcluster, "Session Out"=w298:T4)  [unwired: 8 out]
        n89 = Build Path(base path=w285, name or relative path=path "../Data/Log_temp_storage/log.jpg") -> (appended path=w283:path)
        n90 = call <vilib>:"IMAQdx Unconfigure Acquisition.vi"("error in"=w299, "Session In"=w298) -> ("error out"=w296:errorcluster, "Session Out"=w297:T4)  [unwired: 8 out]
        n91 = call <vilib>:"IMAQdx Close Camera.vi"("error in"=w296, "Session In"=w297) -> ("error out"=w289:errorcluster)  [unwired: 9 out]
        n92 = call-poly "IMAQ Write File 2"("error in (no error)"=w289, "File Path"=w283, "Image"=w286) -> ("error out"=w288:errorcluster)  [unwired: 7 in, 1 out]
        n93 = local write "Tab Control"(enum32{"Page 1", "Page 2", "Page 3", "Page 4"}."Page 2" ("Tab Control")) -> ()
        n94 = call "Imaq Dispose"("Image"=w286, "error in (no error)"=w288) -> ("error out"=w287:errorcluster)  [unwired: 4 in]
        n95 = Bundle By Name(cluster=w290, "IMAQdx Session"=T4 refnum) -> (w291:T5)
        n96 = call <vilib>:"Add State(s) to Queue__JKI_lib_State_Machine.vi"("State(s) in Front (\"\")"="Face ID: Image Processing", "State(s) in (\"\")"=w301) -> ("States Out"=w300:string)  [unwired: 13 in]
      }
      frame "Face ID: Image Processing" {
        n97 = Open Python Session(python version="3.10", python path=path "C:/Users/obiwa/AppData/Local/Programs/Python/Python310/python.exe" ("Python path"), 3:w315) -> (session out=w313:refnum<k35>, error out=w314:errorcluster)
        n98 = Current VI's Path() -> (path=w304:path)
        n99 = Build Path(base path=w304, name or relative path=path "../Python Code/compare_faces_py.py") -> (appended path=w302:path)
        n100 = node ("Python Node")(w313, w302, "find_face_encodings", w314, TRUE) -> (w309:refnum<k35>, w308:errorcluster, w311:bool)  [unwired: 2 out]
        n101 = Close Python Session(session in=w309, error in=w308) -> (11:w307:errorcluster)
        n102 = case shown="True" w311 {
          tunnel: ["Face ID: Initialize Grab Image" "Face ID: Control Panel"] -> w305
          frame False {
            n103 = local write "Tab Control"(enum32{"Page 1", "Page 2", "Page 3"}."Page 1" ("Tab Control")) -> ()
            n104 = Two Button Dialog(message="Login Failed! Please try again to use the app.") -> ()  [unwired: 2 in, 1 out]
          }
          frame True {
            n105 = local write "Tab Control"(enum32{"Page 1", "Page 2", "Page 3", "Page 4"}."Page 3" ("Tab Control")) -> ()
            n106 = One Button Dialog(message="Login Successful! Now you can use the app") -> ()  [unwired: 1 in, 1 out]
          }
        }
        n107 = call <vilib>:"Add State(s) to Queue__JKI_lib_State_Machine.vi"("State(s) in Front (\"\")"=w305, "State(s) in (\"\")"=w319) -> ("States Out"=w318:string)  [unwired: 13 in]
      }
      frame "Face ID: Control Panel" {
        # "Sciezki wzgledne!!!!!!!"
        n108 = Current VI's Path() -> (path=w336:path)
        n109 = event shown="[2] \"Back to userpage\": Value Change" {
          selector: _ -> [_ _ _ _]
          dyn-events: _ -> [_ _ _ _]
          timeout: _ -> [_ _ _ _]
          tunnel: [_ _ _ "Add User: Input Image Init"] -> w331
          tunnel: "Settings Button" -> [_ _ _ _]
          tunnel: "Add user" -> [_ _ _ _]
          tunnel: "Back to userpage" -> [_ _ _ _]
          event Timeout {
            n110 = event-data() -> ()  [unwired: 1 in, 3 out]
          }
          event "Settings Button": Value Change {
            n111 = event-data() -> ()  [unwired: 1 in, 6 out]
          }
          event "Back to userpage": Value Change {
            n112 = event-data() -> ()  [unwired: 1 in, 6 out]
            n113 = local write "Tab Control"(enum32{"Page 1", "Page 2", "Page 3", "Page 4"}."Page 3" ("Tab Control")) -> ()
          }
          event "Add user": Value Change {
            n114 = event-data() -> ()  [unwired: 1 in, 6 out]
            n115 = local write "Tab Control"(enum32{"Page 1", "Page 2", "Page 3", "Page 4"}."Page 4" ("Tab Control")) -> ()
          }
        }
        n116 = Build Path(base path=w336, name or relative path=path "../Python Code") -> (appended path=→"Current VI":path)
        n117 = call <vilib>:"Add State(s) to Queue__JKI_lib_State_Machine.vi"("State(s) in Front (\"\")"=w331, "State(s) in (\"\")"=w332) -> ("States Out"=w333:string)  [unwired: 13 in]
      }
      frame "----------- Control -----------" {
      }
      frame "Control Panel: Add User" {
        n118 = Unbundle By Name(w347) -> ()  [unwired: 1 out]
      }
      frame "-------------- Add User ----------" {
      }
      frame "Add User: Input Image Init" {
        n119 = call "List Available Cameras.vi"("error in"=w359) -> ("error out"=w369:errorcluster, "VendorName"=w370:string[], "Available Cameras"=w371:string[])  [unwired: 8 in]
        n120 = call "Select Camera Dialog.vi"("error in (no error)"=w369, "Vendor Name"=w370, "Camera Name"=w371) -> ("error out"=w365:errorcluster, "No camera?"=w368:bool, "Interface Name"=w367:string)  [unwired: 6 in]
        n121 = case shown="False" w368 {
          tunnel: w367 -> [w382 _]
          tunnel: [w380 T4 refnum ("Session Out")] -> w366
          tunnel: w365 -> [w378 w387]
          tunnel: [w377 w387] -> w358
          tunnel: [w373 w385] -> w364
          tunnel: [w375 T1 refnum ("New Image")] -> w363
          tunnel: ["Add User: Grab Input Image" ("Remaining States") w385] -> w362
          tunnel: [10 w384] -> w356
          tunnel: w361 -> [_ w384]
          tunnel: w360 -> [w373 _]
          frame False {
            w383 = u32 5  # Number of Buffers
            # "{eby nam nie zatrzymaB si w \", \"Event Structure\", \"Idle\" generujemy Timeout"
            # "Musimy stworzy referencj dla przechowywania obrazu w pamici komputera."
            n122 = call <vilib>:"IMAQdx Open Camera.vi"("error in"=w378, "Session In"=w382) -> ("error out"=w379:errorcluster, "Session Out"=w381:T4)  [unwired: 1 in, 7 out]
            n123 = call <vilib>:"IMAQdx Configure Grab.vi"("error in"=w379, "Number of Buffers"=w383, "Session In"=w381) -> ("error out"=w377:errorcluster, "Session Out"=w380:T4)  [unwired: 7 in]
            n124 = call "IMAQ Create"("Image Name"="Acquire Most Recent Image") -> ("New Image"=w375:T1)  [unwired: 3 in, 2 out]
          }
          frame True {
            w385 = ""
            # "Kasujemy kolejne stany.\n! I tak \"idzie\" do \"Error Handler\"."
            # "Generuje bBd: -1074360311"
            # "Camera not found"
          }
        }
        n125 = Bundle By Name(cluster=w355, "New Image"=w363, "IMAQdx Session"=w366) -> (w354:T5)
        n126 = call <vilib>:"Add State(s) to Queue__JKI_lib_State_Machine.vi"("State(s) in Front (\"\")"=w362, "State(s) in (\"\")"=w364) -> ("States Out"=w357:string)  [unwired: 13 in]
      }
      frame "Add User: Grab Input Image" {
        # "Rejestrujemy obrazy...\nPrzetwarzanie obrazów mo|na doda tutaj albo stworzy osobny stan."
        n127 = Unbundle By Name(w402) -> ("IMAQdx Session"=w409:T4, "New Image"=w408:T1)
        n128 = call "Take Image Case Struct.vi"("error in (no error)"=w400, "OK Button"="OK Button 2", "Image In"=w408, "Session In"=w409) -> ("error out"=w399:errorcluster, "f"=w394:string, "Image Out"=w406:T1, "Session Out"=w407:T4)  [unwired: 4 in]
        "Image Display 2" <- w406
        n129 = Concatenate Strings("String", "String 2", ".jpg") -> (w396:string)
        n130 = Equal?(x=w394, y="Face ID: Stop Grab Image") -> (x = y?=w392:bool)
        n131 = Bundle By Name(cluster=w402, "IMAQdx Session"=w407, "New Image"=w406, "Img Path"=w396) -> (w403:T5)
        n132 = Select(t="Add User: Stop Grab Image", s=w392, f="Add User: Grab Input Image") -> (s? t:f=w389:string)
        n133 = call <vilib>:"Add State(s) to Queue__JKI_lib_State_Machine.vi"("State(s) in Front (\"\")"=w389, "State(s) in (\"\")"=w401) -> ("States Out"=w404:string)  [unwired: 13 in]
      }
      frame "Add User: Stop Grab Image" {
        # "WyBczamy Timeout"
        # "Sukces! Wykryli[my twarz, lecimy dalej!"
        n134 = Current VI's Path() -> (path=w423:path)
        n135 = Unbundle By Name(w420) -> ("Img Path"=w414:string, "New Image"=w424:T1, "IMAQdx Session"=w428:T4)
        n136 = Concatenate Strings("..\\Data\\Registered_Users\\", w414) -> (w412:string)
        n137 = String To Path(string=w412) -> (path=w411:path)
        n138 = call <vilib>:"IMAQdx Stop Acquisition.vi"("Session In"=w428) -> ("error out"=w432:errorcluster, "Session Out"=w431:T4)  [unwired: 1 in, 8 out]
        n139 = call <vilib>:"IMAQdx Unconfigure Acquisition.vi"("error in"=w432, "Session In"=w431) -> ("error out"=w429:errorcluster, "Session Out"=w430:T4)  [unwired: 8 out]
        n140 = Build Path(base path=w423, name or relative path=w411) -> (appended path=w422:path)
        n141 = call <vilib>:"IMAQdx Close Camera.vi"("error in"=w429, "Session In"=w430) -> ("error out"=w426:errorcluster)  [unwired: 9 out]
        n142 = call-poly "IMAQ Write File 2"("error in (no error)"=w426, "File Path"=w422, "Image"=w424) -> ("error out"=w425:errorcluster)  [unwired: 7 in, 1 out]
        n143 = call "Imaq Dispose"("Image"=w424, "error in (no error)"=w425) -> ("error out"=w418:errorcluster)  [unwired: 4 in]
        n144 = Bundle By Name(cluster=w420, "IMAQdx Session"=T4 refnum) -> (w416:T5)
        n145 = call <vilib>:"Add State(s) to Queue__JKI_lib_State_Machine.vi"("State(s) in Front (\"\")"="Control Panel: Add User", "State(s) in (\"\")"=w419) -> ("States Out"=w415:string)  [unwired: 13 in]
      }
    }
  }
